vi "infoStepMini.vi"(8 "error in (no error)":errorcluster, 11 "StepList":T1) -> (0 "error out":errorcluster, 3 "Info Test":string)   [LabVIEW 2019]
doc: "Riassume le informazioni principali degli step in un formato più leggibile e ridotto"
uses:
  TypeDef/Step.ctl
  TypeDef/Asset.ctl
  ByteGSAPIBase.lvclass
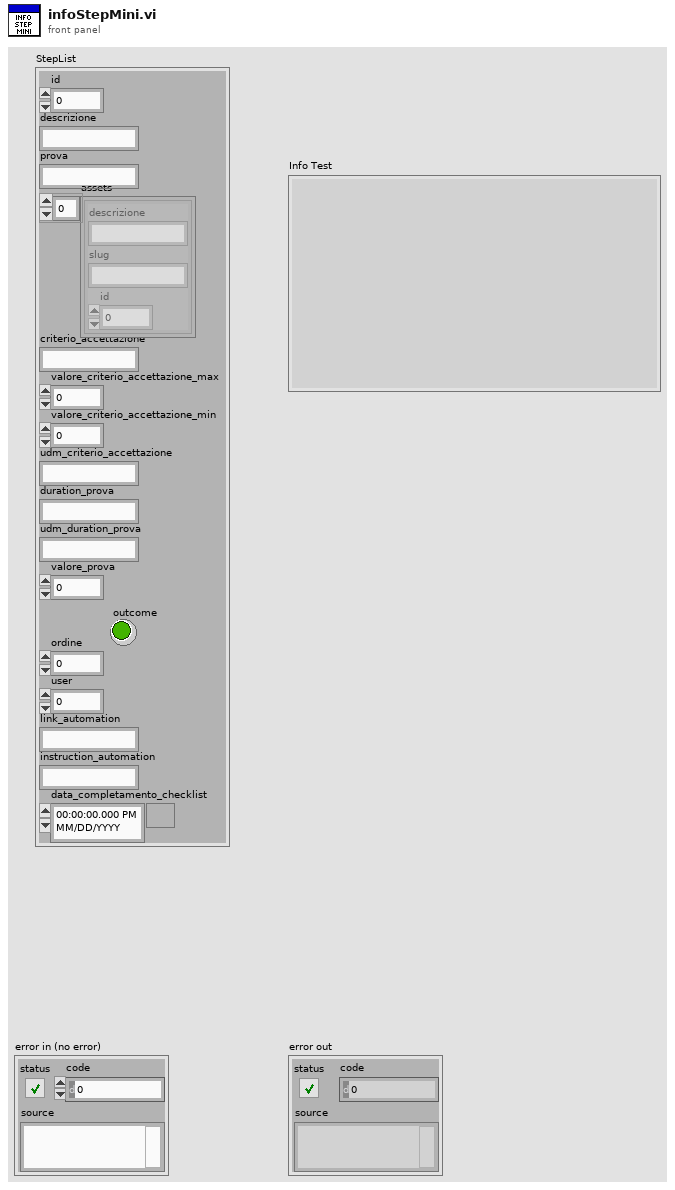
[diagram p1: front panel]
types:
  T1 = typedef "ByteGSWebAPI.lvlib/ByteGSAPIBase.lvclass/Step.ctl" = cluster{"id":i32, "descrizione":string, "prova":string, "assets":T2[], "criterio_accettazione":string, "valore_criterio_accettazione_max":dbl, "valore_criterio_accettazione_min":dbl, "udm_criterio_accettazione":string, "duration_prova":string, "udm_duration_prova":string, "valore_prova":dbl, "ordine":i32, "user":i32, "link_automation":string, "instruction_automation":string, "data_completamento_checklist":timestamp, "outcome":bool}
  T2 = typedef "ByteGSWebAPI.lvlib/ByteGSAPIBase.lvclass/Asset.ctl" = cluster{"descrizione":string, "slug":string, "id":i32}
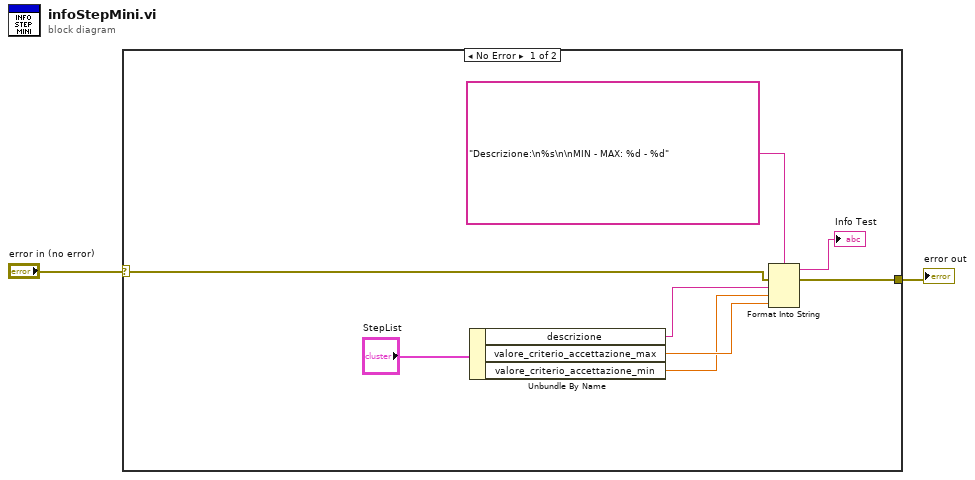
[diagram p0: block diagram]
diagram:
  n1 = case shown="No Error" "error in (no error)" {
    selector: "error in (no error)" -> [w7 w11]
    tunnel: [w6 w11] -> w1
    frame No Error {
      n2 = Unbundle By Name("StepList") -> ("descrizione"=w8:string, "valore_criterio_accettazione_max"=w4:dbl, "valore_criterio_accettazione_min"=w3:dbl)
      n3 = Format Into String(format string="Descrizione:\n%s\n\nMIN - MAX: %d - %d", error in=w7, w8, w3, w4) -> (resulting string=→"Info Test":string, error out=w6:errorcluster)  [unwired: 1 in]
    }
    frame Error {
    }
  }
  "error out" <- w1
